vi "Send + Receive.vi"(0 "comm interface in":refnum<class "Pixy Com.lvclass">, 5 "type":u8, 7 "payload":u8[](array[numeric]), 9 "expected response":u8, 11 "error in":errorcluster, 12 "timeout (ms)":i32=100) -> (4 "comm interface out":refnum<class "Pixy Com.lvclass">, 6 "received":u8[](array[numeric]), 15 "error out":errorcluster)   [LabVIEW 2018, in "Pixy2.lvlib"]
uses:
  Pixy2.lvlib
  Interface/Pixy Com.lvclass
panel:
  out "received":u8[](array[numeric])
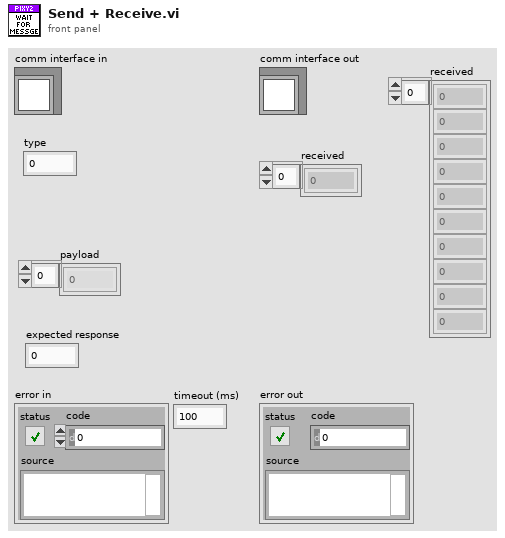
[diagram p1: front panel]
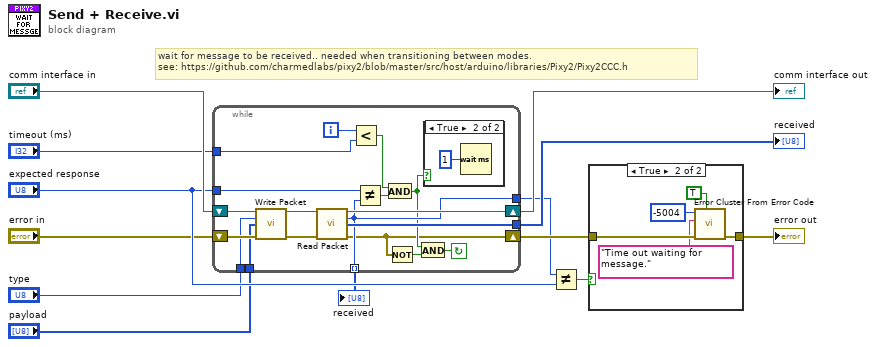
[diagram p0: block diagram]
diagram:
  # "wait for message to be received.. needed when transitioning between modes.\nsee: https://github.com/charmedlabs/pixy2/blob/master/src/host/arduino/libraries/Pixy2/Pixy2CCC.h"
  n1 = while {
    tunnel: [w30] -> w12
    shift-right: [w31] -> w11
    shift-left: "comm interface in" -> [w24]
    shift-right: [w14] -> w10
    shift-left: "error in" -> [w22]
    tunnel: [w18] -> w9
    tunnel: "expected response" -> [w26]
    tunnel: "timeout (ms)" -> [w25]
    tunnel: "payload" -> [w20]
    tunnel: "type" -> [w19]
    tunnel: [w18] -> w1 mode=indexing
    i -> [w29]
    stop <- w17 continue-if-true
    n2 = call "Write Packet.vi"("comm interface in"=w24, "type"=w19, "payload"=w20, "error in"=w22) -> ("comm interface out"=w21:refnum<class "Pixy Com.lvclass">, "error out"=w23:errorcluster)  [unwired: 10 in]
    n3 = call "Read Packet.vi"("comm interface in"=w21, "error in"=w23) -> ("comm interface out"=w31:refnum<class "Pixy Com.lvclass">, "type"=w18:u8, "received"=w30:u8[], "error out"=w14:errorcluster)  [unwired: 10 in]
    n4 = Less?(x=w29, y=w25) -> (x < y?=w27:bool)
    n5 = Not Equal?(x=w26, y=w18) -> (x != y?=w28:bool)
    n6 = And(x=w27, y=w28) -> (x .and. y?=w16:bool)
    n7 = Not(x=w14) -> (.not. x?=w15:bool)
    n8 = And(x=w16, y=w15) -> (x .and. y?=w17:bool)
    n9 = case shown="True" w16 {
      frame False {
      }
      frame True {
        n10 = Wait (ms)(milliseconds to wait=u32 1) -> ()  [unwired: 1 out]
      }
    }
  }
  "received" <- w12
  "comm interface out" <- w11
  "received" <- w1
  n11 = Not Equal?(x=w9, y="expected response") -> (x != y?=w7:bool)
  n12 = case shown="True" w7 {
    tunnel: w10 -> [w33 w38]
    tunnel: [w33 w37] -> w6
    frame False {
    }
    frame True {
      n13 = call <vilib>:"Error Cluster From Error Code.vi"("show call chain? (False)"=TRUE, "error in (no error)"=w38, "error message (\"\")"="Time out waiting for message." ("error message (\"\")"), "error code (0)"=-5004) -> ("error out"=w37:errorcluster)  [unwired: 5 in]
    }
  }
  "error out" <- w6
